vi "proj_utworz_plansze.vi"(10 "Ilosc min":i32=9, 11 "Wielkosc planszy":i32) -> (0 "initialized array":i32[][](array[numeric]), 1 "Maksymalna ilosc \nmin dla danej \nwielkosci planszy":i32, 2 "Komunikaty":string, 3 "Plansza":i32[][](array[numeric]))   [LabVIEW 2020]
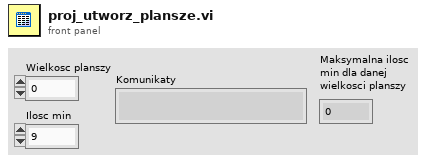
[diagram p1: front panel]
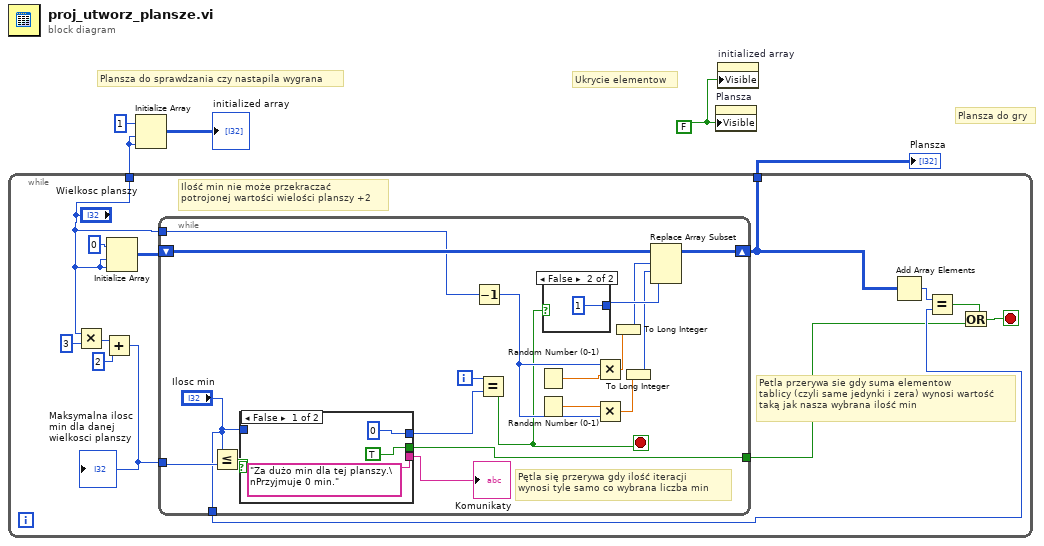
[diagram p0: block diagram]
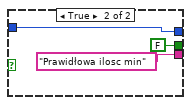
[diagram p2: hidden frame]
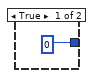
[diagram p3: hidden frame]
diagram:
  w1 = FALSE ("Visible")
  # "Plansza do sprawdzania czy nastapila wygrana"
  # "Plansza do gry"
  # "Ukrycie elementow"
  n1 = while {
    tunnel: [w11] -> w5
    tunnel: ["Wielkosc planszy"] -> w3
    stop <- w6 stop-if-true
    # "Ilość min nie może przekraczać \npotrojonej wartości wielości planszy +2"
    # "Petla przerywa sie gdy suma elementow \ntablicy (czyli same jedynki i zera) wynosi wartość\ntaką jak nasza wybrana ilość min"
    n2 = Multiply(x="Wielkosc planszy", y=3) -> (x*y=w14:i32)
    n3 = Add(x=w14, y=2) -> (x+y=w12:i32)
    "Maksymalna ilosc \nmin dla danej \nwielkosci planszy" <- w12
    n4 = Initialize Array(0, "Wielkosc planszy", "Wielkosc planszy") -> (w17:i32[][])
    n5 = while {
      shift-right: [w36] -> w11
      shift-left: w17 -> [w35]
      tunnel: w12 -> [w24]
      tunnel: ["Ilosc min"] -> w10
      tunnel: "Wielkosc planszy" -> [w21]
      tunnel: [w19] -> w8
      i -> [w26]
      stop <- w20 stop-if-true
      # "Pętla się przerywa gdy ilość iteracji\nwynosi tyle samo co wybrana liczba min"
      n6 = Less Or Equal?(x="Ilosc min", y=w24) -> (x <= y?=w27:bool)
      n7 = case shown="False" w27 {
        tunnel: [0 ("Wielkosc planszy") w42] -> w25
        tunnel: ["Za dużo min dla tej planszy.\nPrzyjmuje 0 min." "Prawidłowa ilosc min"] -> w23
        tunnel: "Ilosc min" -> [_ w42]
        tunnel: [TRUE FALSE] -> w19
        frame False {
        }
        frame True {
        }
      }
      "Komunikaty" <- w23
      n8 = Decrement(x=w21) -> (x-1=w28:i32)
      n9 = Equal?(x=w26, y=w25) -> (x = y?=w20:bool)
      n10 = Random Number (0-1)() -> (number: 0 to 1=w32:dbl)
      n11 = Random Number (0-1)() -> (number: 0 to 1=w31:dbl)
      n12 = case shown="False" w20 {
        tunnel: [0 1] -> w37
        frame True {
        }
        frame False {
        }
      }
      n13 = Multiply(x=w28, y=w32) -> (x*y=w33:dbl)
      n14 = Multiply(x=w31, y=w28) -> (x*y=w34:dbl)
      n15 = To Long Integer(number=w33) -> (32bit integer=w29:i32)
      n16 = To Long Integer(number=w34) -> (32bit integer=w30:i32)
      n17 = Replace Array Subset(array=w35, new element=w37, index (row)=w29, index (col)=w30) -> (w36:i32[][])
    }
    n18 = Add Array Elements(numeric array=w11) -> (sum=w16:i32)
    n19 = Equal?(x=w16, y=w10) -> (x = y?=w7:bool)
    n20 = Or(x=w7, y=w8) -> (x .or. y?=w6:bool)
  }
  "Plansza" <- w5
  n21 = Initialize Array(1 ("element"), w3, w3) -> (→"initialized array":i32[][])
  n22 = property on="Plansza" class="Arr (strict)"("Visible"=w1) -> ()  [unwired: 2 in, 2 out]
  n23 = property on="initialized array" class="Arr (strict)"("Visible"=w1) -> ()  [unwired: 2 in, 2 out]
